vi "Disconnect.vi"(8 "error in (no error)":errorcluster, 11 "NI Vision Camera in":refnum<class "NI Vision Camera.lvclass">) -> (0 "error out":errorcluster, 3 "NI Vision Camera out":refnum<class "NI Vision Camera.lvclass">)   [LabVIEW 2014, in "NI Vision Camera.lvclass"]
uses:
  NI Vision Camera.lvclass
  NI Vision Camera.lvclass/NI Vision Camera.ctl
  <vilib>/vision/driver/NI_Vision_Acquisition_Software.lvlib
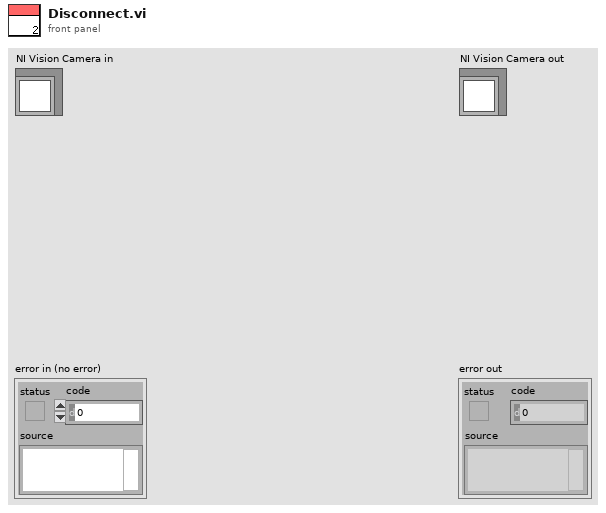
[diagram p1: front panel]
types:
  T1 = typedef "IMAQdx.ctl" = refnum<k21>
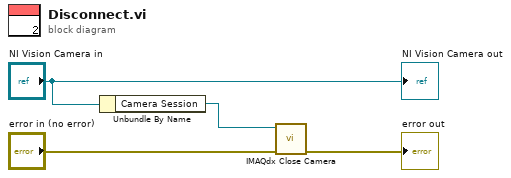
[diagram p0: block diagram]
diagram:
  n1 = Unbundle By Name("NI Vision Camera in") -> ("Camera Session"=w2:T1)
  n2 = call <vilib>:"IMAQdx Close Camera.vi"("error in"="error in (no error)", "Session In"=w2) -> ("error out"=→"error out":errorcluster)  [unwired: 9 in]
  "NI Vision Camera out" <- "NI Vision Camera in"
